vi "SIFS_ReadStatus.vi"(8 "error in":errorcluster, 10 "ID":string, 11 "VISA resource name":refnum<visa-resource-name>) -> (0 "Running when true":bool, 1 "Switch 1 Home":bool, 2 "Switch 2 Homing":bool, 3 "Switch 3":bool, 5 "Status Word":bool[](array[boolean]), 6 "error out":errorcluster)   [LabVIEW 2012]
panel:
  out "read buffer":string
  out "output 4":string
  out "output 3":string
  out "output 2":string
  out "output 1":string
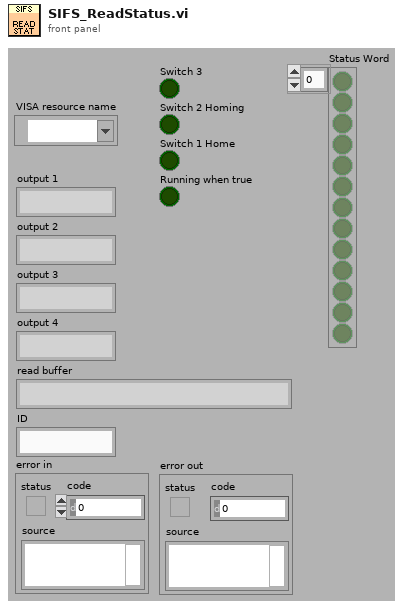
[diagram p1: front panel]
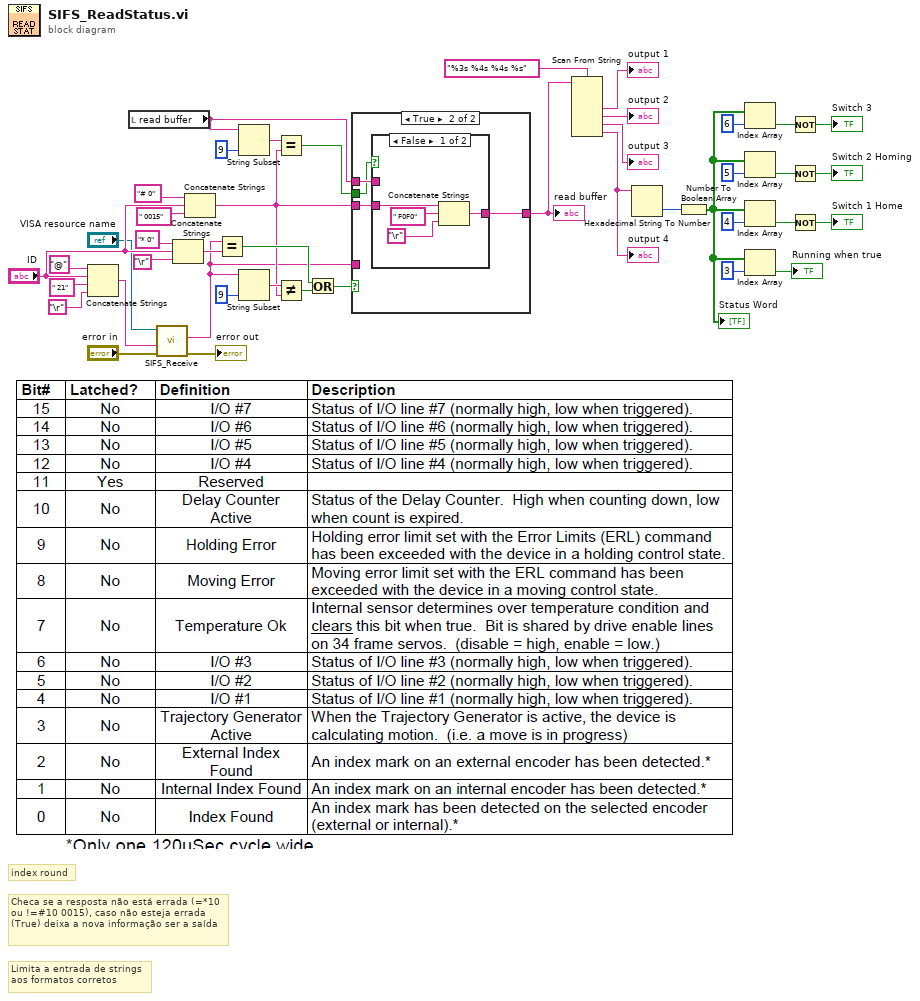
[diagram p0: block diagram]
diagram:
  # "index round"
  # "Checa se a resposta não está errada (=*10 ou !=#10 0015), caso não esteja errada (True) deixa a nova informação ser a saída"
  # "Limita a entrada de strings\naos formatos corretos"
  n1 = Concatenate Strings("@" ("string"), "ID", " 21", "\r") -> (w4:string)
  n2 = local read "read buffer"() -> (w21:string)
  n3 = call "SIFS_Receive.vi"("error in"="error in", "Command to SIFS"=w4, "VISA resource name"="VISA resource name") -> ("error out"=→"error out":errorcluster, "Response from SIFS"=w1:string)  [unwired: 1 in, 2 out]
  n4 = Concatenate Strings("* 0" ("string"), "ID", "\r") -> (w19:string)
  n5 = Concatenate Strings("# 0" ("string"), "ID", " 0015") -> (w8:string)
  n6 = Equal?(x=w1, y=w19) -> (x = y?=w16:bool)
  n7 = String Subset(string=w21, length (rest)=9 ("length (rest)")) -> (substring=w23:string)  [unwired: 1 out]
  n8 = String Subset(string=w1, length (rest)=9 ("length (rest)")) -> (substring=w17:string)  [unwired: 1 out]
  n9 = Equal?(x=w23, y=w8) -> (x = y?=w22:bool)
  n10 = Not Equal?(x=w17, y=w8) -> (x != y?=w15:bool)
  n11 = Or(x=w16, y=w15) -> (x .or. y?=w14:bool)
  n12 = case shown="True" w14 {
    tunnel: [w44 w48] -> w13
    tunnel: w22 -> [_ w46]
    tunnel: w21 -> [_ w47]
    tunnel: w1 -> [w44 _]
    tunnel: w8 -> [_ w45]
    frame False {
    }
    frame True {
      n13 = case shown="False" w46 {
        tunnel: [w52 w53] -> w48
        tunnel: w47 -> [_ w53]
        tunnel: w45 -> [w49 _]
        frame False {
          n14 = Concatenate Strings(w49, " F0F0", "\r") -> (w52:string)
        }
        frame True {
        }
      }
    }
  }
  "read buffer" <- w13
  n15 = Scan From String(format string="%3s %4s %4s %s", input string=w13) -> (output 1=→"output 1":string, output 2=→"output 2":string, output 3=→"output 3":string, output 4=w32:string)  [unwired: 2 in, 7 out]
  "output 4" <- w32
  n16 = Hexadecimal String To Number(string=w32) -> (number=w41:u32)  [unwired: 3 out]
  n17 = Number To Boolean Array(number=w41) -> (Boolean array=w37:bool[])
  "Status Word" <- w37
  n18 = Index Array(array=w37, index=6) -> (element=w31:bool)
  n19 = Index Array(array=w37, index=5) -> (element=w30:bool)
  n20 = Index Array(array=w37, index=4) -> (element=w29:bool)
  n21 = Index Array(array=w37, index=3) -> (element=→"Running when true":bool)
  n22 = Not(x=w31) -> (.not. x?=→"Switch 3":bool)
  n23 = Not(x=w30) -> (.not. x?=→"Switch 2 Homing":bool)
  n24 = Not(x=w29) -> (.not. x?=→"Switch 1 Home":bool)
